vi "_Veritech_LVCM_Provider_InitItems.vi"(8 "error in (no error)":errorcluster, 11 "Items Array":T1[](array[typedef])) -> (0 "error out":errorcluster)   [LabVIEW 2014]
uses:
  <resource>/Framework/Providers/API/ItemRef.ctl
  Support/Utilites/GCMLog/LogInfo.vi
  Support/Utilites/GCMLog/GCMLog.lvclass
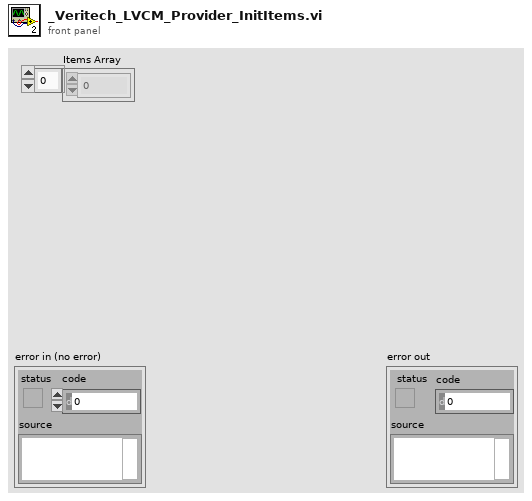
[diagram p1: front panel]
types:
  T1 = typedef "ItemRef.ctl" = u64
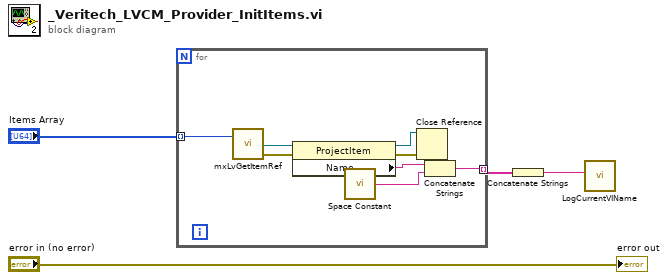
[diagram p0: block diagram]
diagram:
  n1 = for {
    tunnel: "Items Array" -> [w12] mode=indexing
    tunnel: [w7] -> w2 mode=indexing
    n2 = call <resource>:"mxLvGetItemRef.vi"("Item"=w12) -> ("Item Refnum"=w10:refnum<vi>, "error out"=w11:errorcluster)  [unwired: 1 in, 1 out]
    n3 = property class="ProjectItem"(reference=w10, error in=w11) -> (reference out=w5:refnum<vi>, error out=w6:errorcluster, "Name"=w8:string)
    n4 = call <vilib>:"Space Constant.vi"() -> ("String"=w9:string)
    n5 = Close Reference(reference=w5, error in (no error)=w6) -> ()  [unwired: 1 out]
    n6 = Concatenate Strings(w8, w9) -> (w7:string)
  }
  n7 = Concatenate Strings(w2) -> (w1:string)
  n8 = call "LogCurrentVIName.vi"("AdditionalInfo"=w1) -> ()  [unwired: 10 in, 1 out]
  "error out" <- "error in (no error)"
